vi "cluster_v03.vi"() -> ()   [LabVIEW 2009]
panel:
  out "x":dbl
  out "XY Graph":cluster{dbl[], dbl[]}(graph)
  in  "stop":bool
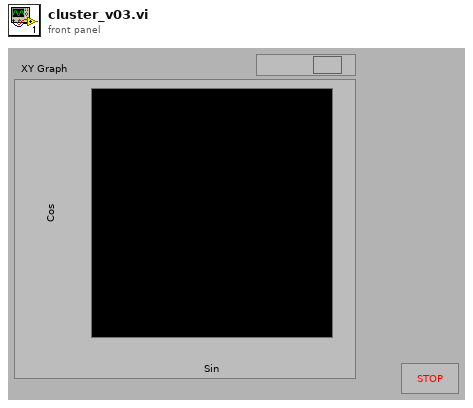
[diagram p1: front panel]
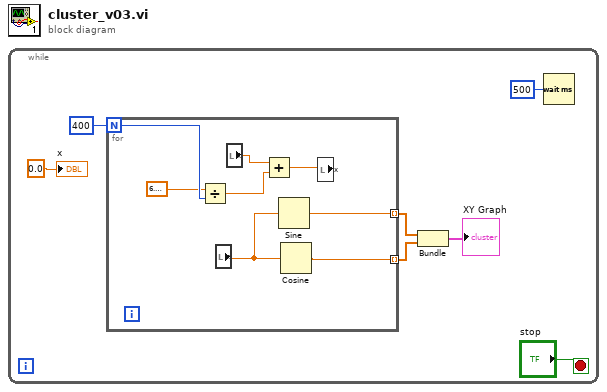
[diagram p0: block diagram]
diagram:
  n1 = while {
    stop <- "stop" stop-if-true
    n2 = for {
      N: 400 -> [w12]
      tunnel: [w15] -> w6 mode=indexing
      tunnel: [w9] -> w4 mode=indexing
      n3 = Divide(x=6.283185307179586, y=w12) -> (x/y=w11:dbl)
      n4 = local read "x"() -> (w10:dbl)
      n5 = local read "x"() -> (w13:dbl)
      n6 = Add(x=w13, y=w11) -> (x+y=w14:dbl)
      n7 = Sine(x=w10) -> (sin(x)=w9:dbl)
      n8 = Cosine(x=w10) -> (cos(x)=w15:dbl)
      n9 = local write "x"(w14) -> ()
    }
    n10 = Bundle(w4, w6) -> (→"XY Graph":cluster{dbl[], dbl[]})  [unwired: 1 in]
    n11 = Wait (ms)(milliseconds to wait=u32 500) -> ()  [unwired: 1 out]
    "x" <- 0.0 ("x")
  }
